vi "Set Slot.vi"(8 "error in":errorcluster, 10 "module":refnum<class "Module.lvclass">, 11 "slot ref in":T2 format="%.0x") -> (0 "error out":errorcluster, 3 "slot ref out":T2 format="%.0x")   [LabVIEW 2017, in "Scan Engine Scripting.lvlib"]
uses:
  Scan Engine Scripting.lvlib
  <vilib>/NI Veristand/Custom Device API/Custom Device Item Ref.ctl
  Modules/Module/Module.lvclass
  Modules.lvlibp/RSI Module/Module Models.ctl
  Modules/NI 9224/NI 9224.lvclass
  Modules.lvlibp/9224/9224.lvclass
  C:/dev/niveristand-scan-engine-ethercat-custom-device/Custom Device Source/Modules.lvlibp/RSI Module/RSI Module.lvclass
  Modules/NI 9228/NI 9228.lvclass
  Modules.lvlibp/9212/9212.lvclass
  Modules/NI 9212/NI 9212.lvclass
  Modules.lvlibp/9213/9213.lvclass
  Modules/NI 9213/NI 9213.lvclass
  Globals/Error Strings.vi
  <vilib>/regexp/Match Regular Expression.xnode
  Modules.lvlibp/RSI Module/RSI Module.lvclass
  Modules.lvlibp
  <vilib>/NI Veristand/Custom Device API/Custom Device API.lvlib
  Scan Engine Custom Device.lvlib
  Modules/Mode Classes/Mode/Mode.lvclass
panel:
  in  "module model":T1
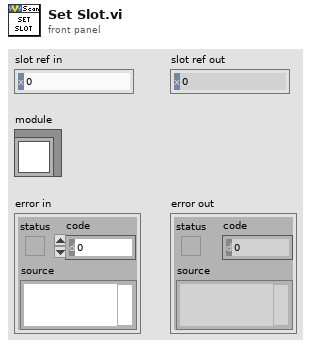
[diagram p1: front panel]
types:
  T1 = typedef "Modules.lvlibp/RSI Module.lvclass/Module Models.ctl" = enum16{"Empty", "NI 9201", "NI 9203", "NI 9205", "NI 9206", "NI 9207", "NI 9208", "NI 9209", "NI 9210", "NI 9211", "NI 9212", "NI 9213", "NI 9214", "NI 9215", "NI 9216", "NI 9217", "NI 9219", "NI 9220", "NI 9221", "NI 9222", "NI 9223", "NI 9224", "NI 9225", "NI 9226", "NI 9227", "NI 9228", "NI 9229", "NI 9233", "NI 9234", "NI 9235", "NI 9236", "NI 9237", "NI 9239", "NI 9242", "NI 9244", "NI 9253", "NI 9263", "NI 9264", "NI 9265", "NI 9266", "NI 9269", "NI 9344", "NI 9350", "NI 9375", "NI 9401", "NI 9402", "NI 9403", "NI 9411", "NI 9421", "NI 9422", "NI 9423", "NI 9425", "NI 9426", "NI 9435", "NI 9436", "NI 9437", "NI 9472", "NI 9474", "NI 9475", "NI 9476", "NI 9477", "NI 9478", "NI 9481", "NI 9482", "NI 9485"}
  T2 = typedef "Custom Device API.lvlib/Custom Device Item Ref.ctl" = u64
  T3 = typedef "Modules.lvlibp/Custom Device API.lvlib/Custom Device Item Ref.ctl" = u64
  T4 = typedef "Modules.lvlibp/RSI Module.lvclass/Slot Settings.ctl" = cluster{"Slot":u32, "EtherCAT?":bool}
  T5 = typedef "Scan Engine Scripting.lvlib/Conversion Time.ctl" = enum16{"High Speed (1k S/s)", "Medium Speed (100 S/s)", "Medium Resolution (50/60Hz Rejection - 12 S/s)", "High Resolution (50/60Hz Rejection - 2 S/s)"}
  T6 = typedef "Scan Engine Scripting.lvlib/Thermocouple Channel.lvclass/Measurement Units.ctl" = enum16{"Raw Volts", "Degrees Kelvin", "Degrees Celsius", "Degrees Fahrenheit", "Degrees Rankine"}
  T7 = typedef "Scan Engine Scripting.lvlib/Thermocouple Channel.lvclass/Thermocouple Type.ctl" = enum16{"J", "K", "T", "E", "R", "S", "N", "B"}
  T8 = typedef "Scan Engine Scripting.lvlib/NI 9212.lvclass/NI 9212 Conversion Time.ctl" = enum16{"High Speed", "Best 60 Hz Rejection", "Best 50 Hz Rejection", "High Resolution"}
  T9 = typedef "Scan Engine Scripting.lvlib/NI 9213.lvclass/NI 9213 Conversion Time.ctl" = enum16{"High Speed", "High Resolution"}
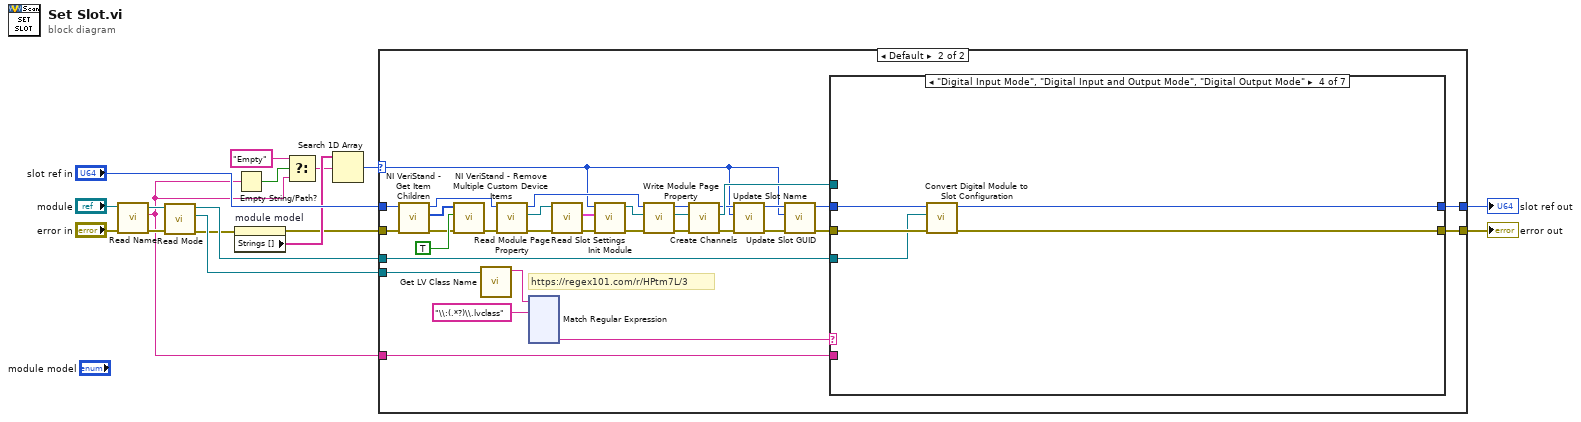
[diagram p0: block diagram]
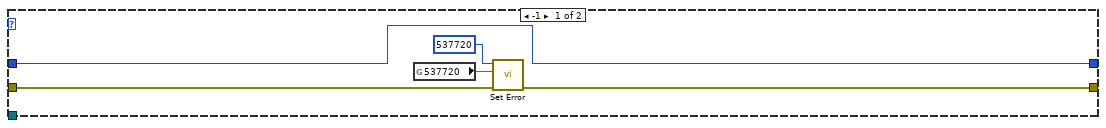
[diagram p2: hidden frame]
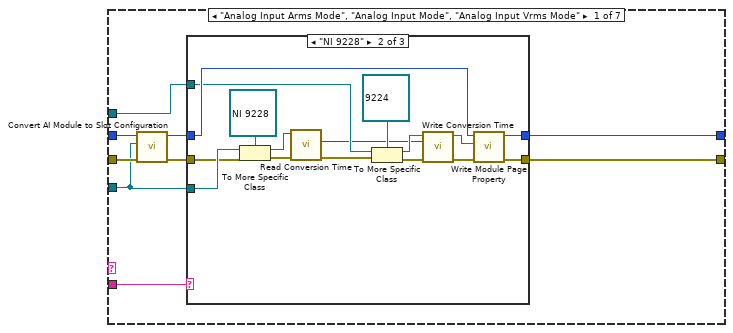
[diagram p3: hidden frame]
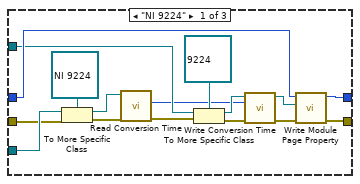
[diagram p4: hidden frame]
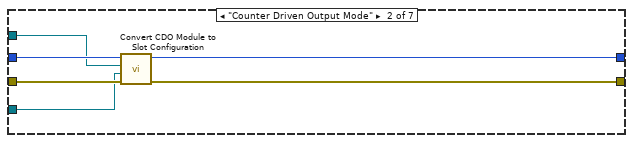
[diagram p6: hidden frame]
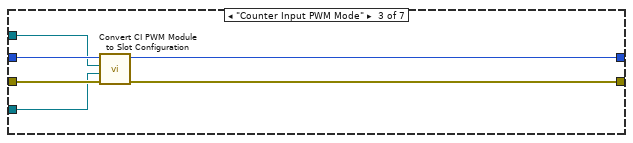
[diagram p7: hidden frame]
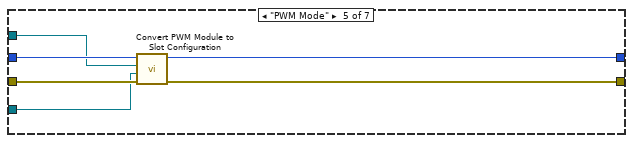
[diagram p8: hidden frame]
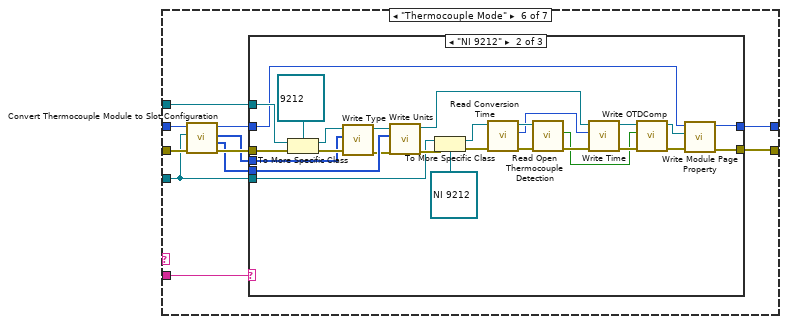
[diagram p9: hidden frame]
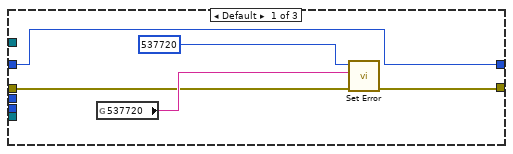
[diagram p10: hidden frame]
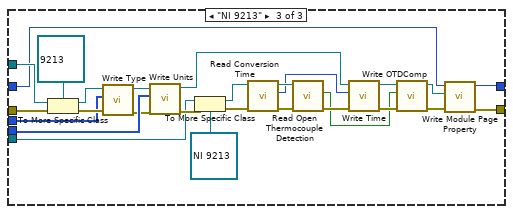
[diagram p11: hidden frame]
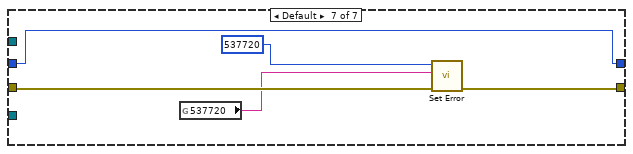
[diagram p12: hidden frame]
diagram:
  n1 = call-dynamic "Read Name.vi"("error in"="error in", "module in"="module") -> ("error out"=w6:errorcluster, "name"=w1:string, "module out"=w5:refnum<class "Module.lvclass">)  [unwired: 7 in]
  n2 = call-dynamic "Read Mode.vi"("error in"=w6, "module in"=w5) -> ("error out"=w2:errorcluster, "mode"=w4:refnum<class "Mode.lvclass">, "module out"=w3:refnum<class "Module.lvclass">)  [unwired: 7 in]
  n3 = property on="module model" class="Enum (strict)"(error in=w2) -> (error out=w12:errorcluster, "Strings []"=w14:string[])  [unwired: 1 in, 1 out]
  n4 = Empty String/Path?(string/path=w1) -> (empty?=w9:bool)
  n5 = Select(t="Empty" ("f"), s=w9, f=w1) -> (s? t:f=w8:string)
  n6 = Search 1D Array(1D array=w14, element=w8) -> (index of element=w13:i32)  [unwired: 1 in]
  n7 = case shown="Default" w13 {
    selector: w13 -> [_ w24]
    tunnel: "slot ref in" -> [w22 w40]
    tunnel: w12 -> [w18 w39]
    tunnel: [w21 w32] -> w16
    tunnel: [w22 w31] -> w15
    tunnel: w4 -> [_ w35]
    tunnel: w3 -> [_ w34]
    tunnel: w1 -> [_ w23]
    frame -1 {
      n8 = global read "Error Strings.vi" "537720"() -> (w19:string)
      n9 = call "Set Error.vi"("error in (no error)"=w18, "Message"=w19, "Code"=537720) -> ("error out"=w21:errorcluster)  [unwired: 8 in]
    }
    frame Default {
      # "https://regex101.com/r/HPtm7L/3"
      n10 = call <vilib>:"NI VeriStand - Get Item Children.vi"("error in (no error)"=w39, "Item Ref in"=w40) -> ("error out"=w46:errorcluster, "Child Refs"=w48:T2[], "Item Ref out"=w45:T2)  [unwired: 6 in, 1 out]
      n11 = call <vilib>:"NI VeriStand - Remove Multiple Custom Device Items.vi"("error in (no error)"=w46, "Force Delete (F)"=TRUE, "Item Refs in"=w48) -> ("error out"=w44:errorcluster)  [unwired: 7 in, 1 out]
      n12 = call <vilib>:"Get LV Class Name.vi"("object"=w35) -> ("class name"=w37:string)  [unwired: 9 in, 1 out]
      n13 = call "Read Module Page Property.vi"("error in (no error)"=w44, "Node Ptr In"=w45) -> ("error out"=w55:errorcluster, "RSI Module"=w54:refnum<class "RSI Module.lvclass">, "Node Ptr Out"=w53:T3)  [unwired: 7 in]
      n14 = xnode "Match Regular Expression"("input string"=w37, "regular expression"="\\:(.*?)\\.lvclass") -> ("submatch 1"=w36:string)  [unwired: 4 in, 5 out]
      n15 = call "Read Slot Settings.vi"("error in (no error)"=w55, "RSI Module in"=w54) -> ("error out"=w52:errorcluster, "Slot Settings"=w51:T4)  [unwired: 7 in, 1 out]
      n16 = call "Init Module.vi"("error in (no error)"=w52, "Slot Settings"=w51, "Module Model"=w24) -> ("error out"=w49:errorcluster, "RSI Module out"=w50:refnum<class "RSI Module.lvclass">)  [unwired: 7 in]
      n17 = call "Write Module Page Property.vi"("error in (no error)"=w49, "RSI Module"=w50, "Node Ptr In"=w53) -> ("error out"=w43:errorcluster, "RSI Module out"=w42:refnum<class "RSI Module.lvclass">, "Node Ptr Out"=w41:T3)  [unwired: 6 in]
      n18 = call-dynamic "Create Channels.vi"("error in (no error)"=w43, "RSI Module in"=w42, "Parent Ref in"=w41) -> ("error out"=w30:errorcluster, "RSI Module out"=w33:refnum<class "RSI Module.lvclass">, "Parent Ref out"=w29:T3)  [unwired: 6 in]
      n19 = call "Update Slot Name.vi"("error in"=w30, "module"=w24, "slot ref in"=w29) -> ("error out"=w28:errorcluster, "slot ref out"=w27:T2)  [unwired: 6 in, 1 out]
      n20 = call "Update Slot GUID.vi"("error in"=w28, "module model"=w24, "slot ref in"=w27) -> ("error out"=w26:errorcluster, "slot ref out"=w25:T2)  [unwired: 7 in]
      n21 = case shown="\"Digital Input Mode\", \"Digital Input and Output Mode\", \"Digital Output Mode\"" w36 {
        tunnel: w34 -> [w174 w215 w222 w227 w232 w239 _]
        tunnel: w26 -> [w179 w220 w225 w231 w237 w248 w310]
        tunnel: w33 -> [w173 w216 w221 _ w233 w245 _]
        tunnel: w25 -> [w180 w217 w226 w228 w234 w247 w312]
        tunnel: [w175 w218 w223 w230 w235 w241 w309] -> w32
        tunnel: [w177 w219 w224 w229 w236 w240 w312] -> w31
        tunnel: w23 -> [w172 _ _ _ _ w238 _]
        frame "Analog Input Arms Mode", "Analog Input Mode", "Analog Input Vrms Mode" {
          n22 = call "Convert AI Module to Slot Configuration.vi"("error in"=w179, "module in"=w174, "slot ref in"=w180) -> ("error out"=w176:errorcluster, "slot ref out"=w178:T2)  [unwired: 7 in]
          n23 = case shown="\"NI 9228\"" w172 {
            tunnel: w178 -> [w188 w204 w214]
            tunnel: [w181 w201 w214] -> w177
            tunnel: w176 -> [w195 w211 w213]
            tunnel: [w182 w202 w213] -> w175
            tunnel: w174 -> [w196 w212 _]
            tunnel: w173 -> [w187 w203 _]
            frame "NI 9224" {
              n24 = To More Specific Class(target class=refnum<class "NI 9224.lvclass"> refnum, reference=w196, error in=w195) -> (specific class reference=w186:refnum<class "NI 9224.lvclass">, error out=w185:errorcluster)
              n25 = call-dynamic "Read Conversion Time.vi"("error in"=w185, "NI 9224 in"=w186) -> ("error out"=w184:errorcluster, "conversion time"=w183:T5)  [unwired: 7 in, 1 out]
              n26 = To More Specific Class(target class=refnum<class "9224.lvclass"> refnum ("9224 in"), reference=w187, error in=w184) -> (specific class reference=w193:refnum<class "9224.lvclass">, error out=w192:errorcluster)
              n27 = call-dynamic "Write Conversion Time.vi"("error in"=w192, "Conversion Time"=w183, "9224 in"=w193) -> ("error out"=w191:errorcluster, "9224 out"=w190:refnum<class "9224.lvclass">)  [unwired: 7 in]
              n28 = call "Write Module Page Property.vi"("error in (no error)"=w191, "RSI Module"=w190, "Node Ptr In"=w188) -> ("error out"=w182:errorcluster, "Node Ptr Out"=w181:T3)  [unwired: 6 in, 1 out]
            }
            frame "NI 9228" {
              n29 = To More Specific Class(target class=refnum<class "NI 9228.lvclass"> refnum, reference=w212, error in=w211) -> (specific class reference=w200:refnum<class "NI 9228.lvclass">, error out=w199:errorcluster)
              n30 = call-dynamic "Read Conversion Time.vi"("error in"=w199, "NI 9228 in"=w200) -> ("error out"=w198:errorcluster, "conversion time"=w197:T5)  [unwired: 7 in, 1 out]
              n31 = To More Specific Class(target class=refnum<class "9224.lvclass"> refnum ("9224 in"), reference=w203, error in=w198) -> (specific class reference=w209:refnum<class "9224.lvclass">, error out=w208:errorcluster)
              n32 = call-dynamic "Write Conversion Time.vi"("error in"=w208, "Conversion Time"=w197, "9224 in"=w209) -> ("error out"=w207:errorcluster, "9224 out"=w206:refnum<class "9224.lvclass">)  [unwired: 7 in]
              n33 = call "Write Module Page Property.vi"("error in (no error)"=w207, "RSI Module"=w206, "Node Ptr In"=w204) -> ("error out"=w202:errorcluster, "Node Ptr Out"=w201:T3)  [unwired: 6 in, 1 out]
            }
            frame Default {
            }
          }
        }
        frame "Counter Driven Output Mode" {
          n34 = call "Convert CDO Module to Slot Configuration.vi"("error in"=w220, "module in"=w215, "RSI Module in"=w216, "slot ref in"=w217) -> ("error out"=w218:errorcluster, "slot ref out"=w219:T2)  [unwired: 6 in]
        }
        frame "Counter Input PWM Mode" {
          n35 = call "Convert CI PWM Module to Slot Configuration.vi"("error in"=w225, "module in"=w222, "RSI Module in"=w221, "slot ref in"=w226) -> ("error out"=w223:errorcluster, "slot ref out"=w224:T2)  [unwired: 6 in]
        }
        frame "Digital Input Mode", "Digital Input and Output Mode", "Digital Output Mode" {
          n36 = call "Convert Digital Module to Slot Configuration.vi"("error in"=w231, "module in"=w227, "slot ref in"=w228) -> ("error out"=w230:errorcluster, "slot ref out"=w229:T2)  [unwired: 7 in]
        }
        frame "PWM Mode" {
          n37 = call "Convert PWM Module to Slot Configuration.vi"("error in"=w237, "module in"=w232, "RSI Module in"=w233, "slot ref in"=w234) -> ("error out"=w235:errorcluster, "slot ref out"=w236:T2)  [unwired: 6 in]
        }
        frame "Thermocouple Mode" {
          n38 = call "Convert Thermocouple Module to Slot Configuration.vi"("error in"=w248, "module in"=w239, "slot ref in"=w247) -> ("error out"=w246:errorcluster, "channel measurement units"=w242:T6[], "channel thermocouple types"=w244:T7[], "slot ref out"=w243:T2)  [unwired: 5 in]
          n39 = case shown="\"NI 9212\"" w238 {
            tunnel: w246 -> [w250 w280 w307]
            tunnel: w245 -> [_ w279 w306]
            tunnel: w244 -> [_ w275 w302]
            tunnel: w243 -> [w253 w274 w301]
            tunnel: w242 -> [_ w273 w300]
            tunnel: [w249 w270 w297] -> w241
            tunnel: [w253 w269 w296] -> w240
            tunnel: w239 -> [_ w265 w292]
            frame Default {
              n40 = global read "Error Strings.vi" "537720"() -> (w251:string)
              n41 = call "Set Error.vi"("error in (no error)"=w250, "Message"=w251, "Code"=537720) -> ("error out"=w249:errorcluster)  [unwired: 8 in]
            }
            frame "NI 9212" {
              n42 = To More Specific Class(target class=refnum<class "9212.lvclass"> refnum ("9213 in"), reference=w279, error in=w280) -> (specific class reference=w276:refnum<class "9212.lvclass">, error out=w278:errorcluster)
              n43 = call-dynamic "Write Type.vi"("error in (no error)"=w278, "Type"=w275, "9213 in"=w276) -> ("error out"=w272:errorcluster, "9213 out"=w271:refnum<class "9212.lvclass">)  [unwired: 7 in]
              n44 = call-dynamic "Write Units.vi"("error in (no error)"=w272, "Units"=w273, "9213 in"=w271) -> ("error out"=w266:errorcluster, "9213 out"=w268:refnum<class "9212.lvclass">)  [unwired: 7 in]
              n45 = To More Specific Class(target class=refnum<class "NI 9212.lvclass"> refnum ("NI 9212 in"), reference=w265, error in=w266) -> (specific class reference=w263:refnum<class "NI 9212.lvclass">, error out=w264:errorcluster)
              n46 = call-dynamic "Read Conversion Time.vi"("error in"=w264, "NI 9212 in"=w263) -> ("error out"=w261:errorcluster, "conversion time"=w260:T8, "NI 9212 out"=w262:refnum<class "NI 9212.lvclass">)  [unwired: 7 in]
              n47 = call-dynamic "Read Open Thermocouple Detection.vi"("error in"=w261, "NI 9212 in"=w262) -> ("error out"=w259:errorcluster, "open thermocouple detection"=w254:bool)  [unwired: 7 in, 1 out]
              n48 = call-dynamic "Write Time.vi"("error in (no error)"=w259, "Conversion Time"=w260, "9213 in"=w268) -> ("error out"=w258:errorcluster, "9213 out"=w257:refnum<class "9212.lvclass">)  [unwired: 7 in]
              n49 = call-dynamic "Write OTDComp.vi"("error in (no error)"=w258, "OTDComp"=w254, "9212 in"=w257) -> ("error out"=w255:errorcluster, "9212 out"=w256:refnum<class "9212.lvclass">)  [unwired: 7 in]
              n50 = call "Write Module Page Property.vi"("error in (no error)"=w255, "RSI Module"=w256, "Node Ptr In"=w274) -> ("error out"=w270:errorcluster, "Node Ptr Out"=w269:T3)  [unwired: 6 in, 1 out]
            }
            frame "NI 9213" {
              n51 = To More Specific Class(target class=refnum<class "9213.lvclass"> refnum ("9213 in"), reference=w306, error in=w307) -> (specific class reference=w303:refnum<class "9213.lvclass">, error out=w305:errorcluster)
              n52 = call-dynamic "Write Type.vi"("error in (no error)"=w305, "Type"=w302, "9213 in"=w303) -> ("error out"=w299:errorcluster, "9213 out"=w298:refnum<class "9213.lvclass">)  [unwired: 7 in]
              n53 = call-dynamic "Write Units.vi"("error in (no error)"=w299, "Units"=w300, "9213 in"=w298) -> ("error out"=w293:errorcluster, "9213 out"=w295:refnum<class "9213.lvclass">)  [unwired: 7 in]
              n54 = To More Specific Class(target class=refnum<class "NI 9213.lvclass"> refnum ("NI 9212 in"), reference=w292, error in=w293) -> (specific class reference=w290:refnum<class "NI 9213.lvclass">, error out=w291:errorcluster)
              n55 = call-dynamic "Read Conversion Time.vi"("error in"=w291, "NI 9213 in"=w290) -> ("error out"=w288:errorcluster, "conversion time"=w287:T9, "NI 9213 out"=w289:refnum<class "NI 9213.lvclass">)  [unwired: 7 in]
              n56 = call "Read Open Thermocouple Detection.vi"("error in"=w288, "NI 9213 in"=w289) -> ("error out"=w286:errorcluster, "open thermocouple detection"=w281:bool)  [unwired: 7 in, 1 out]
              n57 = call-dynamic "Write Time.vi"("error in (no error)"=w286, "Conversion Time"=w287, "9213 in"=w295) -> ("error out"=w285:errorcluster, "9213 out"=w284:refnum<class "9213.lvclass">)  [unwired: 7 in]
              n58 = call-dynamic "Write OTDComp.vi"("error in (no error)"=w285, "OTDComp"=w281, "9213 in"=w284) -> ("error out"=w282:errorcluster, "9213 out"=w283:refnum<class "9213.lvclass">)  [unwired: 7 in]
              n59 = call "Write Module Page Property.vi"("error in (no error)"=w282, "RSI Module"=w283, "Node Ptr In"=w301) -> ("error out"=w297:errorcluster, "Node Ptr Out"=w296:T3)  [unwired: 6 in, 1 out]
            }
          }
        }
        frame Default {
          n60 = global read "Error Strings.vi" "537720"() -> (w308:string)
          n61 = call "Set Error.vi"("error in (no error)"=w310, "Message"=w308, "Code"=537720) -> ("error out"=w309:errorcluster)  [unwired: 8 in]
        }
      }
    }
  }
  "error out" <- w16
  "slot ref out" <- w15
